vi "FMS Data Array.vi"(11 "Game Data":string) -> (0 "FMS Data Array":string[](array[string]), 2 "Scale":string, 3 "Switch":string)   [LabVIEW 2017]
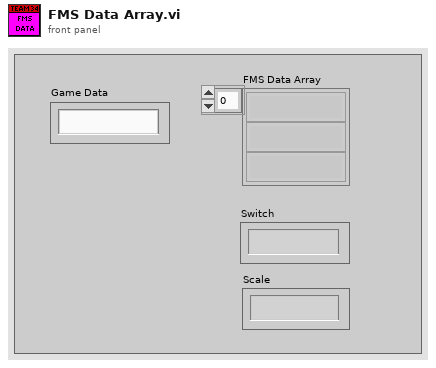
[diagram p1: front panel]
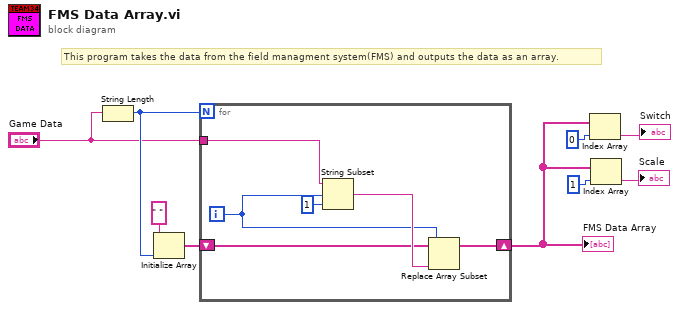
[diagram p0: block diagram]
diagram:
  # "This program takes the data from the field managment system(FMS) and outputs the data as an array."
  n1 = String Length(string="Game Data") -> (length=w9:i32)
  n2 = Initialize Array(" ", w9) -> (w7:string[])
  n3 = for {
    N: w9 -> [_]
    shift-right: [w12] -> w4
    shift-left: w7 -> [w13]
    tunnel: "Game Data" -> [w10]
    i -> [w11]
    n4 = String Subset(string=w10, offset (0)=w11, length (rest)=1 ("length (rest)")) -> (substring=w14:string)
    n5 = Replace Array Subset(array=w13, new element=w14, index=w11) -> (w12:string[])
  }
  "FMS Data Array" <- w4
  n6 = Index Array(array=w4, index=0) -> (element=→"Switch":string)
  n7 = Index Array(array=w4, index=1) -> (element=→"Scale":string)
